vi "Shoot Manual and Auto Management Vr2.vi"(0 "Auto Preparation for Shooting":bool, 1 "Le Fire At Will":bool, 2 "override \"Ready to Fire\"":bool, 5 "Pilot X":dbl, 7 "Pilot Y":dbl, 9 "Elevation":dbl, 11 "Shoot Motors":dbl, 12 "Stop Centerizing":bool, 13 "ReCenterize":bool, 14 "Fine Tune":bool) -> (6 "X Drive Arcade":dbl, 10 "Y Drive Arcade":dbl, 15 "Ready to Fire!":bool)   [LabVIEW 2012]
uses:
  Motors Values.vi
  BotStatus.vi
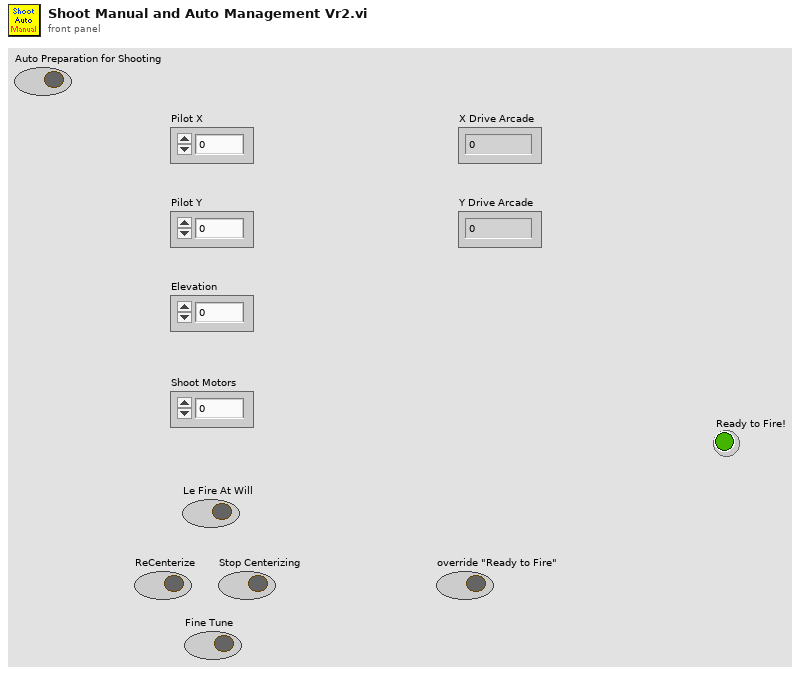
[diagram p1: front panel]
types:
  T1 = typedef "WPI_EncoderDevRef.ctl" = cluster{"DevStatus":errorcluster, "EncoderIndex":T2, "CounterIndex":T3, "DistancePerCount":dbl, "Decoding Type":T4}
  T2 = typedef "FPGA_EncoderIdx.ctl" = enum8{"Enc 0", "Enc 1", "Enc 2", "Enc 3", "Invalid"}
  T3 = typedef "FPGA_CounterCtrSystemIndex.ctl" = enum8{"Ctr 0", "Ctr 1", "Ctr 2", "Ctr 3", "Ctr 4", "Ctr 5", "Ctr 6", "Ctr 7", "Invalid"}
  T4 = typedef "WPI_EncoderType.ctl" = enum16{"1x", "2x", "4x"}
  T5 = typedef "WPI_ServoDeviceRef.ctl" = cluster{"DeviceStatus":errorcluster, "Digital Module":T6, "PWM Channel":T7, "DeadBand":T8}
  T6 = typedef "FPGA_TypedefDigitalModule.ctl" = enum16{"Digital Module 1", "Digital Module 2"}
  T7 = typedef "FPGA_DIOPWMChannel.ctl" = enum8{"PWM 1", "PWM 2", "PWM 3", "PWM 4", "PWM 5", "PWM 6", "PWM 7", "PWM 8", "PWM 9", "PWM 10", "Invalid"}
  T8 = typedef "WPI_PWMDeadband.ctl" = cluster{"Name":string, "maxPositivePwm":i32, "minPositivePwm":i32, "centerPwm":i32, "maxNegativePwm":i32, "minNegativePwm":i32, "angularRange":u16}
  T9 = cluster{"Middle":bool, "InCannon":bool, "InFlipper":bool, "FlipperAtPlace":bool, "Bottom":bool, "FrisbeeDirection":bool}
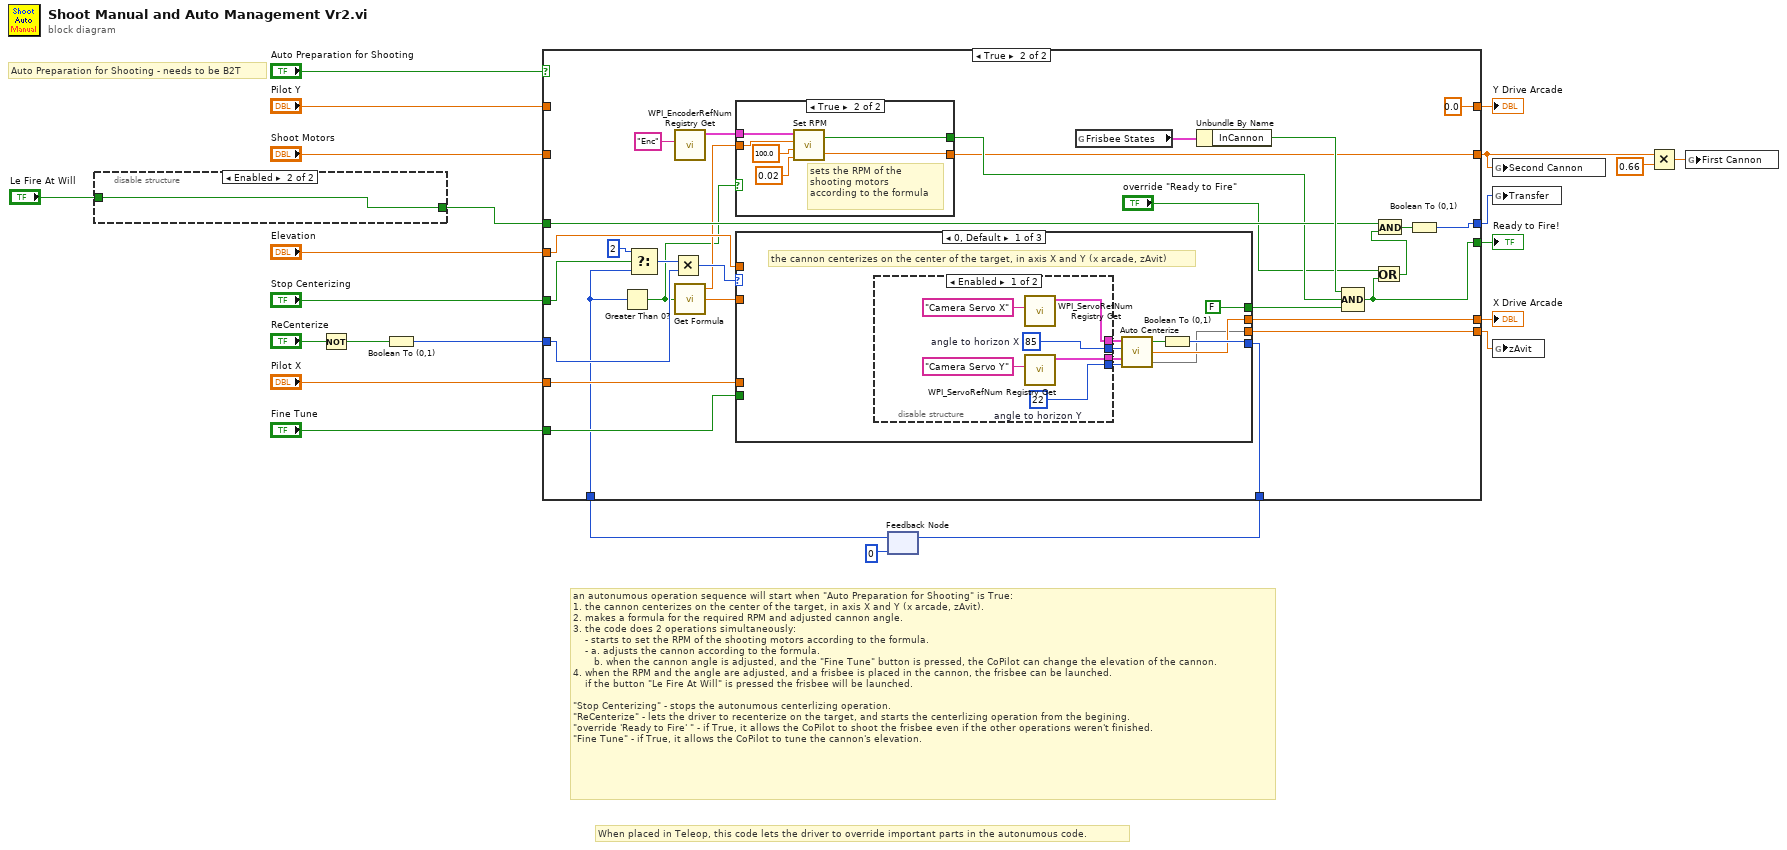
[diagram p0: block diagram]
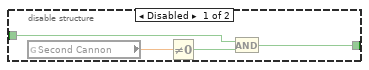
[diagram p2: hidden frame]
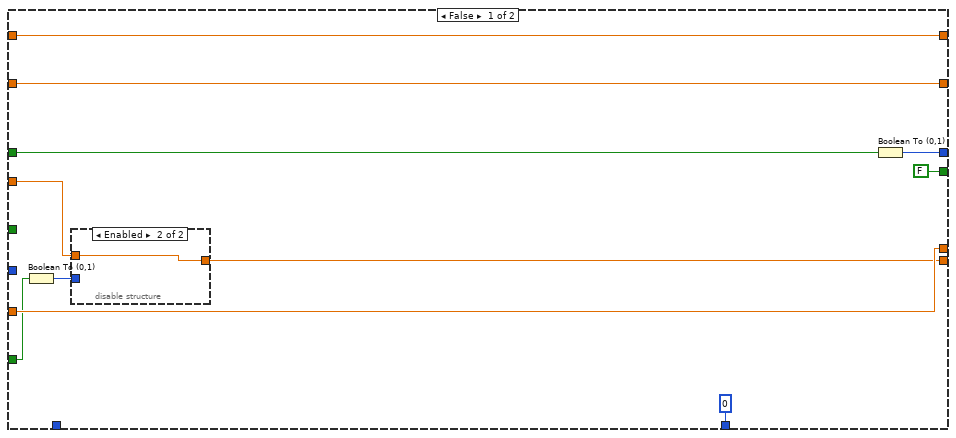
[diagram p3: hidden frame]
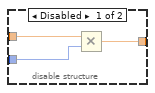
[diagram p4: hidden frame]
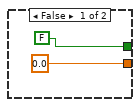
[diagram p5: hidden frame]
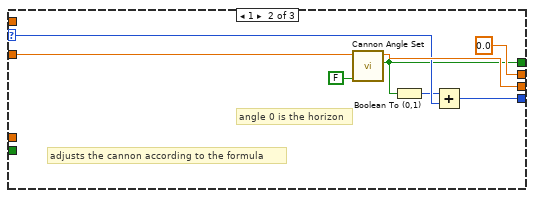
[diagram p7: hidden frame]
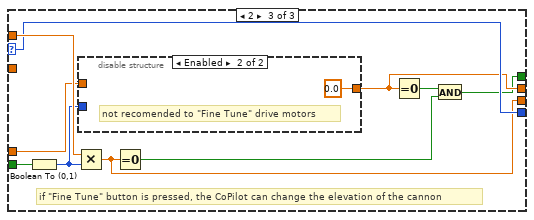
[diagram p8: hidden frame]
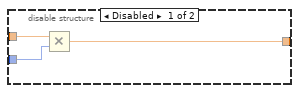
[diagram p9: hidden frame]
diagram:
  # "When placed in Teleop, this code lets the driver to override important parts in the autonumous code."
  # "an autonumous operation sequence will start when \"Auto Preparation for Shooting\" is True:\n1. the cannon centerizes on the center of the target, in axis X and Y (x arcade, zAvit).\n2. makes a formula for the required RPM and adjusted cannon angle.\n3. the code does 2 operations simultaneously:\n    - starts to set the RPM of the shooting motors according to the formula.\n    - a. adjusts the cannon according to the formula.\n       b. when the cannon angle is adjusted, and the \"Fine Tune\" button is pressed, the CoPilot can change the elevation of the cannon.\n4. when the RPM and the angle are adjusted, and a frisbee is placed in the cannon, the frisbee can be launched.\n    if the button \"Le Fire At Will\" is pressed the frisbee will be launched.\n\n\"Stop Centerizing\" - stops the autonumous centerlizing operation.\n\"ReCenterize\" - lets the driver to recenterize on the target, and starts the centerlizing operation from the begining.\n\"override 'Ready to Fire' \" - if True, it allows the CoPilot to shoot the frisbee even if the other operations weren't finished.\n\"Fine Tune\" - if True, it allows the CoPilot to tune the cannon's elevation."
  # "Auto Preparation for Shooting - needs to be B2T"
  n1 = disable-structure shown="Enabled" {
    disable-tunnel: "Le Fire At Will" -> [w25 w28]
    disable-tunnel: [w24 w28] -> w9
    frame Disabled {
      n2 = global read "Motors Values.vi" "Second Cannon"() -> (w27:dbl)
      n3 = Not Equal To 0?(x=w27) -> (x != 0?=w26:bool)
      n4 = And(x=w25, y=w26) -> (x .and. y?=w24:bool)
    }
    frame Enabled {
    }
  }
  n5 = Not(x="ReCenterize") -> (.not. x?=w5:bool)
  n6 = Boolean To (0,1)(Boolean=w5) -> (0, 1=w4:i16)
  n7 = feedback #1(0) -> (w2:i32)
  n8 = case shown="True" "Auto Preparation for Shooting" {
    tunnel: [w34 w64] -> w20
    tunnel: [w39 w65] -> w21
    tunnel: "Pilot X" -> [w39 w60]
    tunnel: "Elevation" -> [w38 w61]
    tunnel: w9 -> [w32 w66]
    tunnel: [w37 w70] -> w18
    tunnel: [w36 w50] -> w15
    tunnel: "Shoot Motors" -> [w36 _]
    tunnel: "Pilot Y" -> [w35 _]
    tunnel: [w35 0.0] -> w12
    tunnel: [FALSE w48] -> w11
    tunnel: "Fine Tune" -> [w30 w62]
    tunnel: "Stop Centerizing" -> [_ w59]
    tunnel: w4 -> [_ w55]
    tunnel: w2 -> [_ w45]
    tunnel: [0 w44] -> w1
    frame False {
      n9 = Boolean To (0,1)(Boolean=w30) -> (0, 1=w33:i16)
      n10 = disable-structure shown="Enabled" {
        disable-tunnel: w38 -> [w42 w43]
        disable-tunnel: [w41 w43] -> w34
        disable-tunnel: w33 -> [w40 _]
        frame Disabled {
          n11 = Multiply(x=w42, y=w40) -> (x*y=w41:dbl)
        }
        frame Enabled {
        }
      }
      n12 = Boolean To (0,1)(Boolean=w32) -> (0, 1=w37:i16)
    }
    frame True {
      n13 = Greater Than 0?(x=w45) -> (x > 0?=w49:bool)
      n14 = Select(t=2, s=w59, f=w45) -> (s? t:f=w56:i32)
      n15 = Multiply(x=w56, y=w55) -> (x*y=w57:i32)
      n16 = call <vilib>:"WPI_EncoderRefNum Registry Get.vi"("refnum name"="Enc") -> ("EncoderDevRef"=w52:T1)  [unwired: 9 in, 1 out]
      n17 = call "Get Formula.vi"("Make Formula"=w49) -> ("Cannon Angle Set Point"=w63:dbl, "RPM Set Point"=w53:dbl)  [unwired: 2 in, 1 out]
      n18 = case shown="True" w49 {
        tunnel: w53 -> [_ w78]
        tunnel: w52 -> [_ w77]
        tunnel: [FALSE ("READY!") w76] -> w51
        tunnel: [0.0 ("Vbus Out") w75] -> w50
        frame False {
        }
        frame True {
          # "sets the RPM of the\nshooting motors\naccording to the formula"
          n19 = call "Set RPM.vi"("Gain Vbus"=0.02, "Range RPM"=100.0, "Set Point RPM"=w78, "EncoderDevRef"=w77) -> ("Vbus Out"=w75:dbl, "READY!"=w76:bool)
        }
      }
      n20 = case shown="0, Default" w57 {
        selector: w57 -> [_ w100 w109]
        tunnel: [w86 0.0 ("X Drive Arcade") w108] -> w65
        tunnel: [w85 w102 w107] -> w64
        tunnel: [w89 w98 w109] -> w44
        tunnel: w63 -> [_ w103 _]
        tunnel: w62 -> [_ _ w113]
        tunnel: w61 -> [_ _ w112]
        tunnel: w60 -> [_ _ w111]
        tunnel: [FALSE ("On Target") w97 w104] -> w54
        frame 0, Default {
          # "the cannon centerizes on the center of the target, in axis X and Y (x arcade, zAvit)"
          n21 = disable-structure shown="Enabled" {
            disable-tunnel: [w94 _] -> w84
            disable-tunnel: [w92 _] -> w83
            disable-tunnel: [w91 _] -> w82
            disable-tunnel: [w90 _] -> w81
            frame Enabled {
              w90 = u16 22  # angle to horizon Y
              w91 = u16 85  # angle to horizon X
              n22 = call <vilib>:"WPI_ServoRefNum Registry Get.vi"("refnum name"="Camera Servo X") -> ("ServoDeviceRef"=w94:T5)  [unwired: 9 in, 1 out]
              n23 = call <vilib>:"WPI_ServoRefNum Registry Get.vi"("refnum name"="Camera Servo Y") -> ("ServoDeviceRef"=w92:T5)  [unwired: 9 in, 1 out]
            }
            frame Disabled {
            }
          }
          n24 = call "Auto Centerize.vi"("angle to horizon Y"=w81, "Camera Y ServoDeviceRef"=w83, "angle to horizon X"=w82, "Camera X ServoDeviceRef"=w84) -> (0:w85, "X Drive Arcade"=w86:dbl, "Centerized?"=w87:bool)
          n25 = Boolean To (0,1)(Boolean=w87) -> (0, 1=w89:i16)
        }
        frame 1 {
          # "adjusts the cannon according to the formula"
          # "angle 0 is the horizon"
          n26 = call "Cannon Angle Set.vi"("set angle 0 to be min angle"=FALSE, "Angle Set Point"=w103) -> ("On Target"=w97:bool, "zAvit Vbus Out"=w102:dbl)  [unwired: 8 in]
          n27 = Boolean To (0,1)(Boolean=w97) -> (0, 1=w99:i16)
          n28 = Add(x=w99, y=w100) -> (x+y=w98:i32)
        }
        frame 2 {
          # "if \"Fine Tune\" button is pressed, the CoPilot can change the elevation of the cannon"
          n29 = Boolean To (0,1)(Boolean=w113) -> (0, 1=w110:i16)
          n30 = Multiply(x=w112, y=w110) -> (x*y=w107:dbl)
          n31 = disable-structure shown="Enabled" {
            disable-tunnel: w111 -> [w116 _]
            disable-tunnel: w110 -> [w115 _]
            disable-tunnel: [w114 0.0] -> w108
            frame Disabled {
              n32 = Multiply(x=w116, y=w115) -> (x*y=w114:dbl)
            }
            frame Enabled {
              # "not recomended to \"Fine Tune\" drive motors"
            }
          }
          n33 = Equal To 0?(x=w107) -> (x = 0?=w106:bool)
          n34 = Equal To 0?(x=w108) -> (x = 0?=w105:bool)
          n35 = And(x=w105, y=w106) -> (x .and. y?=w104:bool)
        }
      }
      n36 = global read "BotStatus.vi" "Frisbee States"() -> (w72:T9)
      n37 = Unbundle By Name(w72) -> ("InCannon"=w71:bool)
      n38 = Compound Arithmetic op=AND(w71, w51, w54) -> (w48:bool)
      n39 = Or(x="override \"Ready to Fire\"", y=w48) -> (x .or. y?=w46:bool)
      n40 = And(x=w66, y=w46) -> (x .and. y?=w67:bool)
      n41 = Boolean To (0,1)(Boolean=w67) -> (0, 1=w70:i16)
    }
  }
  "X Drive Arcade" <- w21
  "Y Drive Arcade" <- w12
  "Ready to Fire!" <- w11
  n42 = feedback-in #1(w1) -> ()
  n43 = global write "Motors Values.vi" "Second Cannon"(w15) -> ()
  n44 = global write "Motors Values.vi" "Transfer"(w18) -> ()
  n45 = global write "Motors Values.vi" "zAvit"(w20) -> ()
  n46 = Multiply(x=w15, y=0.66) -> (x*y=w16:dbl)
  n47 = global write "Motors Values.vi" "First Cannon"(w16) -> ()
